vi "OCR_TrainBOX.vi"(8 "error in (no error)":errorcluster, 10 "exp#":string, 11 "lang.font.exp":string) -> (0 "error out":errorcluster, 2 "standard error":string[](array[string]), 3 "standard output":string[](array[string]))   [LabVIEW 2019]
uses:
  Controls/cmd.ctl
panel:
  out "error":bool
  # "eng1.segoe.exp1.tr"
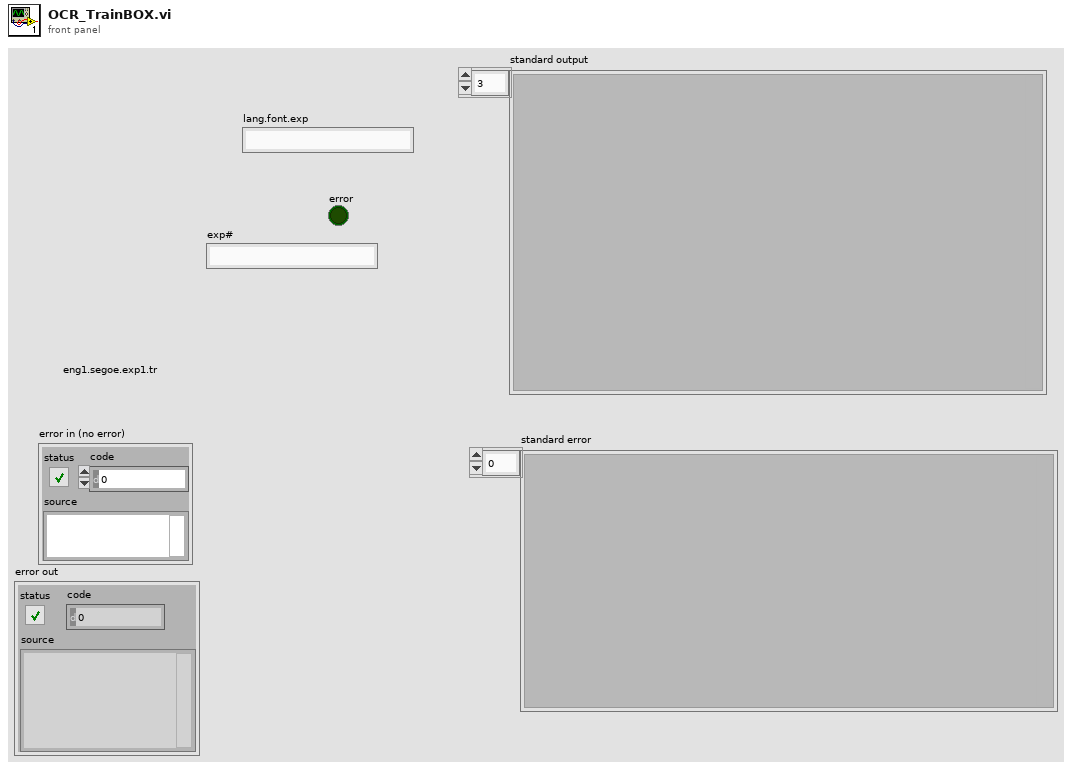
[diagram p1: front panel]
types:
  T1 = typedef "cmd.ctl" = enum16{"Box Train", "unicharset", "ShapeTable", "mftraining1", "mftraining2", "cntraining", "rename", "move files", "combine"}
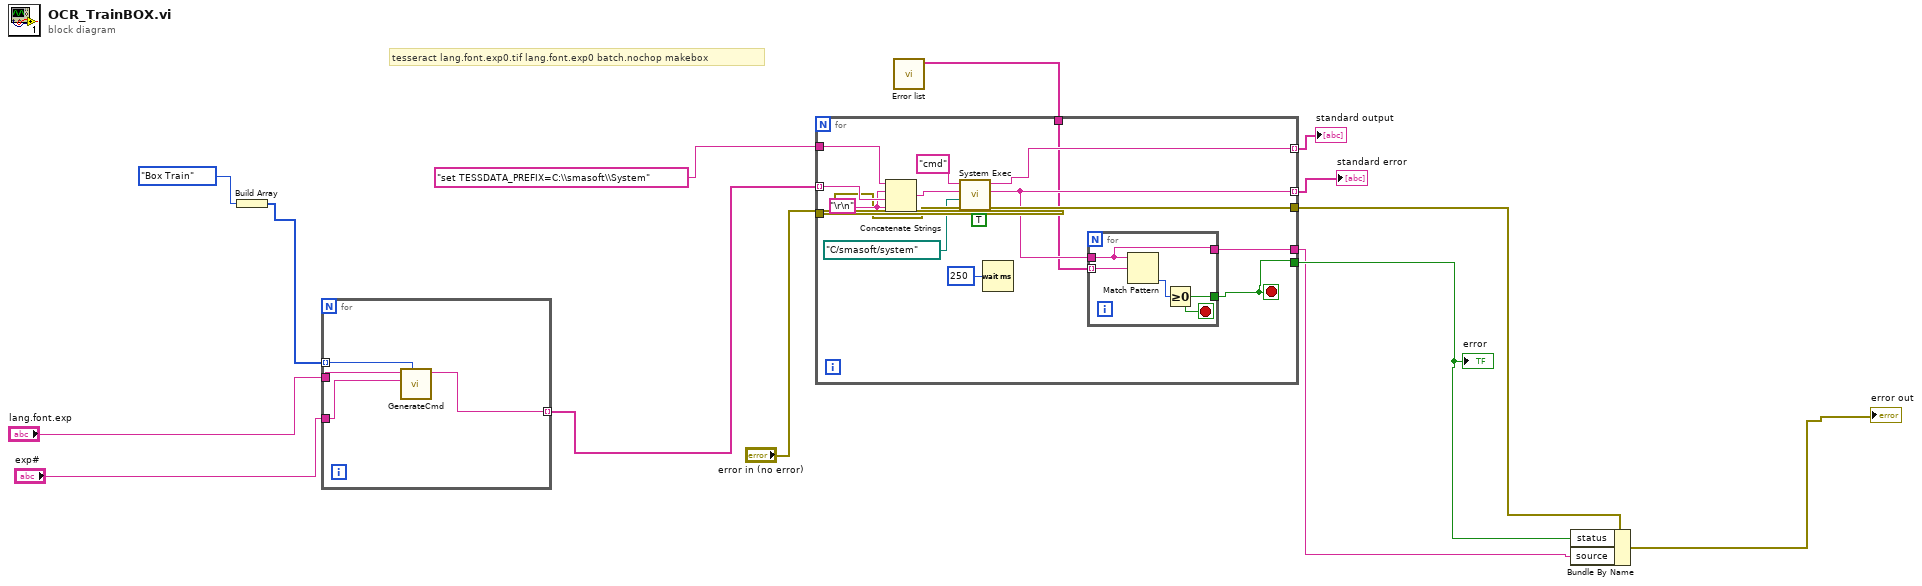
[diagram p0: block diagram]
diagram:
  # "tesseract lang.font.exp0.tif lang.font.exp0 batch.nochop makebox"
  n1 = Build Array(cmd."Box Train" ("Cmd")) -> (w4:T1[])
  n2 = for {
    tunnel: w4 -> [w18] mode=indexing
    tunnel: "lang.font.exp" -> [w17]
    tunnel: "exp#" -> [w16]
    tunnel: [w15] -> w12 mode=indexing
    n3 = call "GenerateCmd.vi"("Cmd"=w18, "exp#"=w16, "lang.font.exp"=w17) -> ("CMD"=w15:string)  [unwired: 7 in, 1 out]
  }
  n4 = call "Error list.vi"() -> ("regular expression"=w2:string[])  [unwired: 11 in]
  n5 = for {
    tunnel: w12 -> [w33] mode=indexing
    tunnel: "set TESSDATA_PREFIX=C:\\smasoft\\System" ("standard input") -> [w31]
    tunnel: "error in (no error)" -> [w26]
    tunnel: [w25] -> w10
    tunnel: [w20] -> w8
    tunnel: [w23] -> w6 mode=indexing
    tunnel: [w22] -> w7 mode=indexing
    tunnel: w2 -> [w21]
    tunnel: [w19] -> w1
    stop <- w20 stop-if-true
    w32 = "\r\n"
    n6 = Concatenate Strings(w31, w32, w33, w32) -> (w30:string)
    n7 = call <vilib>:"System Exec.vi"("run minimized? (F)"=TRUE, "error in (no error)"=w26, "working directory"=path "C:/smasoft/system", "standard input"=w30, "command line"="cmd") -> ("error out"=w25:errorcluster, "standard error"=w23:string, "standard output"=w22:string)  [unwired: 3 in, 1 out]
    n8 = Wait (ms)(milliseconds to wait=u32 250) -> ()  [unwired: 1 out]
    n9 = for {
      tunnel: w23 -> [w35]
      tunnel: w21 -> [w37] mode=indexing
      tunnel: [w35] -> w19
      tunnel: [w34] -> w20
      stop <- w34 stop-if-true
      n10 = Match Pattern(string=w35, regular expression=w37) -> (offset past match=w36:i32)  [unwired: 1 in, 3 out]
      n11 = Greater Or Equal To 0?(x=w36) -> (x >= 0?=w34:bool)
    }
  }
  "error" <- w8
  "standard output" <- w7
  "standard error" <- w6
  n12 = Bundle By Name(cluster=w10, "status"=w8, "source"=w1) -> (→"error out":errorcluster)
